vi "SQL操作.vi"() -> ()   [LabVIEW 2017]
panel:
  out "连接的字符串 2":string
  in  "WorkNumber Delete":string
  out "连接的字符串":string
  in  "TestMessage":string
  in  "ProductNumber":string
  in  "WorkNumber":string
  out "Data":string[][](array[string])
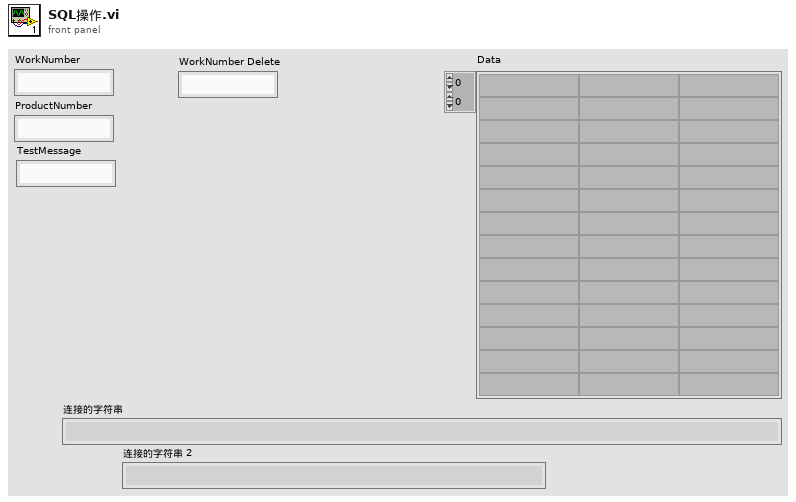
[diagram p1: front panel]
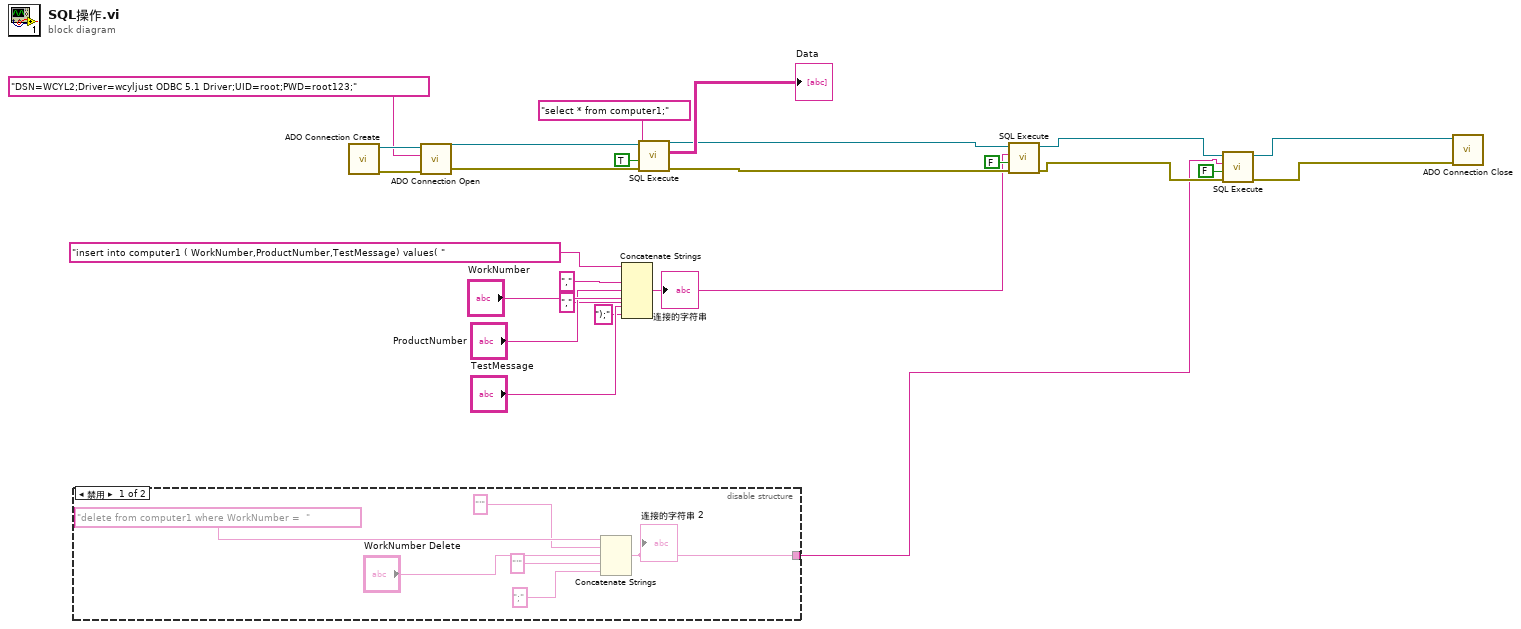
[diagram p0: block diagram]
diagram:
  n1 = disable-structure shown="禁用" {
    disable-tunnel: [w28 _] -> w1
    frame Disabled {
      n2 = Concatenate Strings("delete from computer1 where WorkNumber =  " ("Command Text"), "'" ("字符串"), "WorkNumber Delete", "'" ("字符串"), ";" ("字符串")) -> (w28:string)
      "连接的字符串 2" <- w28
    }
    frame Enabled {
    }
  }
  n3 = call <userlib>:"ADO Connection Create.vi"() -> ("error out"=w17:errorcluster, "ADODB._Connection Out"=w18:refnum<k7>)  [unwired: 10 in]
  n4 = call <userlib>:"ADO Connection Open.vi"("error in (no error)"=w17, "ConnectionString"="DSN=WCYL2;Driver=wcyljust ODBC 5.1 Driver;UID=root;PWD=root123;", "ADODB._Connection In"=w18) -> ("error out"=w14:errorcluster, "ADODB._Connection Out"=w15:refnum<k7>)  [unwired: 7 in]
  n5 = Concatenate Strings("insert into computer1 ( WorkNumber,ProductNumber,TestMessage) values( " ("Command Text"), "WorkNumber", "," ("字符串"), "ProductNumber", "," ("字符串"), "TestMessage", ");" ("字符串")) -> (w7:string)
  "连接的字符串" <- w7
  n6 = call <userlib>:"SQL Execute.vi"("error in (no error)"=w14, "Return Data (T)"=TRUE, "Command Text"="select * from computer1;", "ADODB._Connection In"=w15) -> ("error out"=w8:errorcluster, "Data"=→"Data":string[][], "ADODB._Connection Out"=w9:refnum<k7>)  [unwired: 4 in, 1 out]
  n7 = call <userlib>:"SQL Execute.vi"("error in (no error)"=w8, "Return Data (T)"=FALSE, "Command Text"=w7, "ADODB._Connection In"=w9) -> ("error out"=w3:errorcluster, "ADODB._Connection Out"=w5:refnum<k7>)  [unwired: 4 in, 2 out]
  n8 = call <userlib>:"SQL Execute.vi"("error in (no error)"=w3, "Return Data (T)"=FALSE, "Command Text"=w1, "ADODB._Connection In"=w5) -> ("error out"=w2:errorcluster, "ADODB._Connection Out"=w4:refnum<k7>)  [unwired: 4 in, 2 out]
  n9 = call <userlib>:"ADO Connection Close.vi"("error in (no error)"=w2, "ADODB._Connection In"=w4) -> ()  [unwired: 8 in, 2 out]
